vi "iWorx - Humidity.vi"() -> ()   [LabVIEW 2012]
uses:
  <vilib>/DAQmx/create/channels.llb/DAQmx Create Channel (AI-Voltage-Basic).vi
  <vilib>/DAQmx/read.llb/DAQmx Read (Analog 1D Wfm NChan 1Samp).vi
  vi.lib/iWorx/iWorx Set Points.ctl
panel:
  in  "Reset Scale":bool
  in  "Stop":bool
  in  "Log Info Button":bool
  in  "Set Up":bool
  in  "Channel":u16(ring) items=["Channel 1", "Channel 2"]
  in  "Pause Button":bool
  in  "Snapshot":bool
  out "Processed Signal":dbl(knob) caption="Relative Humidity" scale=0.0..100.0
  out "Waveform Chart":waveform(dbl)(graph)
  in  "Sample Timing":u16(ring)=200 items=["20Hz"=50, "5 Hz"=200, "2 Hz"=500, "1 Hz"=1000, ".5 Hz"=2000, ".2 Hz"=5000]
  in  "Clear Chart":bool
  in  "Open Log":bool
  in  "Rescale Y":bool
  out "Raw Signal":dbl(knob) scale=-5.0..5.0
  # "iWorx - Humidity - Data Logger"
  # "Sensor Input"
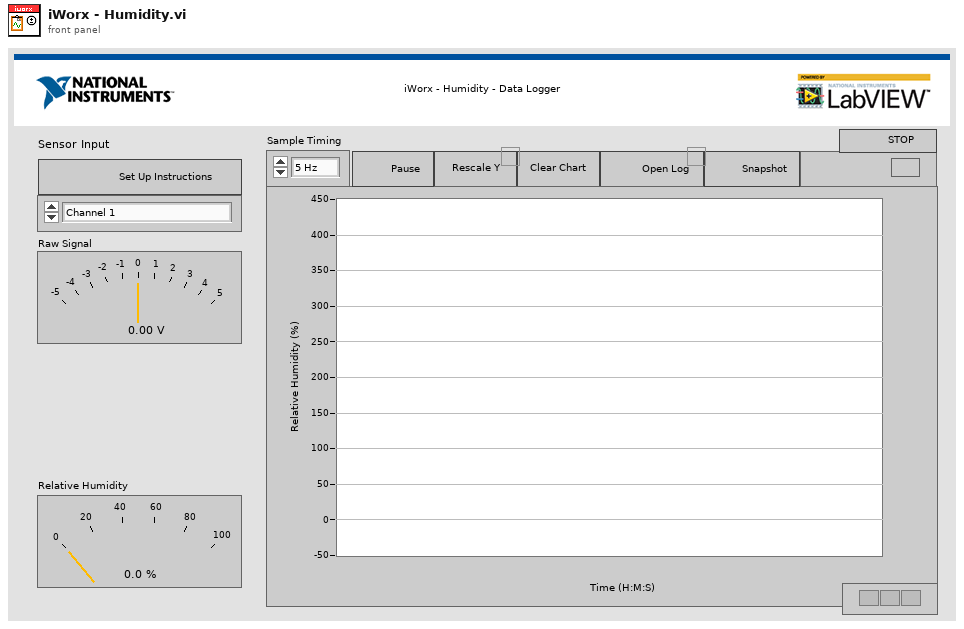
[diagram p1: front panel]
types:
  T1 = typedef "iWorx Set Points.ctl" = cluster{"SP1 Voltage":dbl, "SP1 Value":dbl, "SP2 Voltage":dbl, "SP2 Value":dbl}
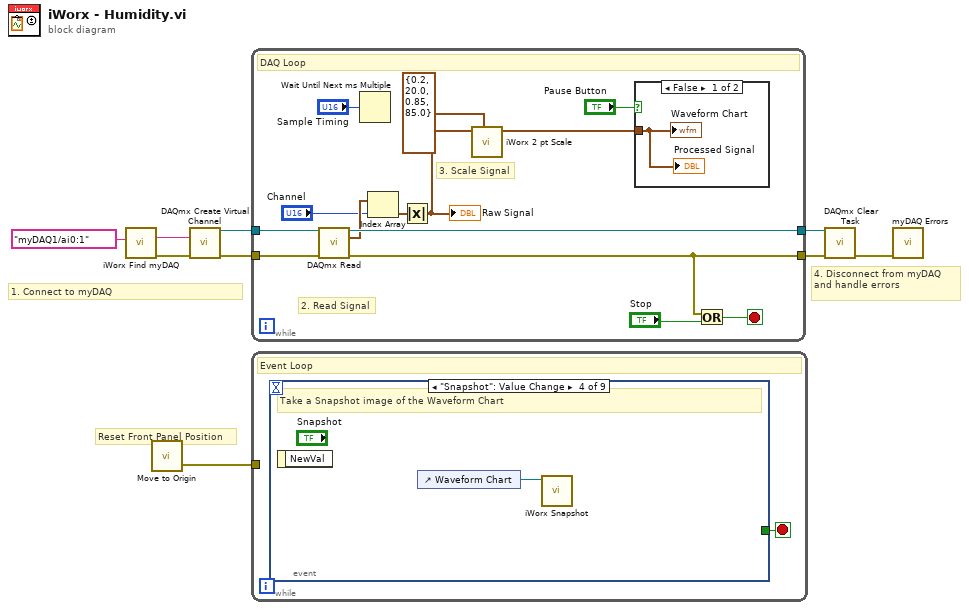
[diagram p0: block diagram]
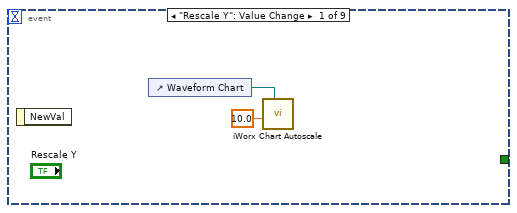
[diagram p2: hidden frame]
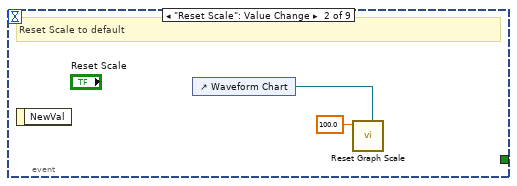
[diagram p3: hidden frame]
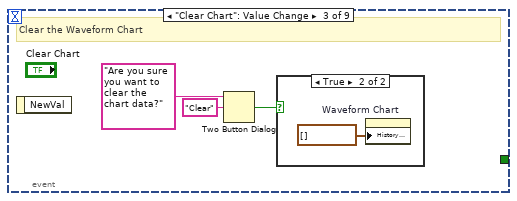
[diagram p4: hidden frame]
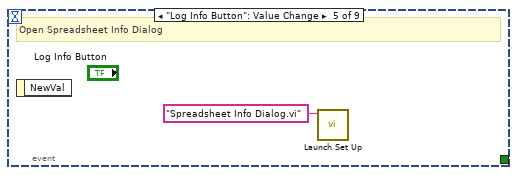
[diagram p6: hidden frame]
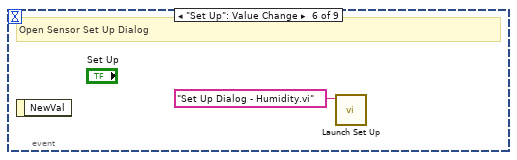
[diagram p7: hidden frame]
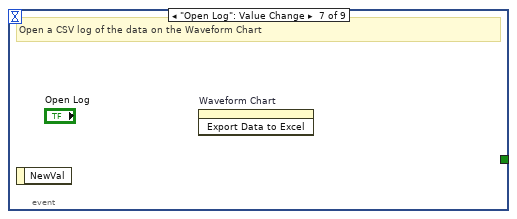
[diagram p8: hidden frame]
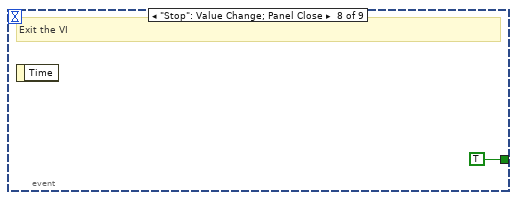
[diagram p9: hidden frame]
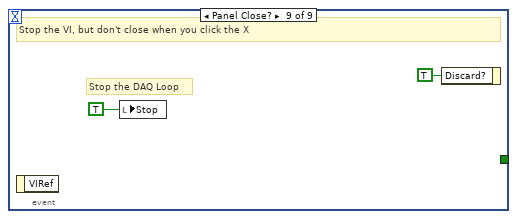
[diagram p10: hidden frame]
diagram:
  # "Reset Front Panel Position"
  # "4. Disconnect from myDAQ and handle errors"
  # "1. Connect to myDAQ"
  n1 = call "iWorx Find myDAQ.vi"("Preferred myDAQ (myDAQ1)"=tag "myDAQ1/ai0:1") -> ("Error Out"=w3:errorcluster, "DAQmx Physical Channel"=w4:tag)  [unwired: 6 in, 3 out]
  n2 = call "Move to Origin.vi"() -> ("Error Out"=w1:errorcluster)  [unwired: 3 in]
  n3 = call-poly <vilib>:"DAQmx Create Virtual Channel.vi"("physical channels"=w4, "error in"=w3) -> ("task out"=w7:refnum<k21>, "error out"=w6:errorcluster)  [unwired: 12 in]
  n4 = while {
    tunnel: w7 -> [w22]
    tunnel: [w21] -> w9
    tunnel: w6 -> [w20]
    tunnel: [w18] -> w8
    stop <- w19 stop-if-true
    # "3. Scale Signal"
    # "2. Read Signal"
    # "DAQ Loop"
    n5 = call-poly <vilib>:"DAQmx Read.vi"("task/channels in"=w22, "error in"=w20) -> ("task out"=w21:refnum<k21>, "data"=w16:waveform(dbl)[], "error out"=w18:errorcluster)  [unwired: 11 in]
    n6 = Wait Until Next ms Multiple(millisecond multiple="Sample Timing") -> ()  [unwired: 1 out]
    n7 = Index Array(array=w16, index="Channel") -> (element=w11:waveform(dbl))
    n8 = Absolute Value(x=w11) -> (abs(x)=w10:waveform(dbl))
    "Raw Signal" <- w10
    n9 = call "iWorx 2 pt Scale.vi"("Set Points"=T1 {"SP1 Voltage"=0.2, "SP1 Value"=20.0, "SP2 Voltage"=0.85, "SP2 Value"=85.0}, "Raw Waveform"=w10) -> ("Scaled Value"=w15:waveform(dbl))  [unwired: 7 in, 2 out]
    n10 = case shown="False" "Pause Button" {
      tunnel: w15 -> [w24 _]
      frame False {
        "Waveform Chart" <- w24
        "Processed Signal" <- w24
      }
      frame True {
        # "Do Not update controls"
      }
    }
    n11 = Or(x=w18, y="Stop") -> (x .or. y?=w19:bool)
  }
  n12 = while {
    tunnel: w1 -> [_]
    stop <- w25 stop-if-true
    # "Event Loop"
    n13 = event shown="[3] \"Snapshot\": Value Change" {
      selector: _ -> [_ _ _ _ _ _ _ _ _]
      dyn-events: _ -> [_ _ _ _ _ _ _ _ _]
      timeout: _ -> [_ _ _ _ _ _ _ _ _]
      tunnel: [_ _ _ _ _ _ _ TRUE _] -> w25
      event "Rescale Y": Value Change {
        n14 = event-data() -> ()  [unwired: 1 in, 1 out]
        n15 = control-ref of="Waveform Chart"() -> (w27:refnum<vi>)
        n16 = call "iWorx Chart Autoscale.vi"("Selection Chart"=w27, "Rounding Multiple (10)"=10.0 ("Rounding Multiple (1)")) -> ()  [unwired: 7 in, 3 out]
      }
      event "Reset Scale": Value Change {
        # "Reset Scale to default"
        n17 = event-data() -> ()  [unwired: 1 in, 1 out]
        n18 = control-ref of="Waveform Chart"() -> (w29:refnum<vi>)
        n19 = call "Reset Graph Scale.vi"("WaveformChart in"=w29, "Maximum (100)"=100.0) -> ()  [unwired: 9 in, 1 out]
      }
      event "Clear Chart": Value Change {
        # "Clear the Waveform Chart"
        n20 = event-data() -> ()  [unwired: 1 in, 1 out]
        n21 = Two Button Dialog(message="Are you sure you want to clear the chart data?", 2:"Clear" ("T button name (\"OK\")")) -> (T button?=w31:bool)  [unwired: 1 in]
        n22 = case shown="True" w31 {
          frame False {
          }
          frame True {
            n23 = property on="Waveform Chart" class="WFChart (strict)"("History Data"=waveform(dbl)[] []) -> ()  [unwired: 2 in, 2 out]
          }
        }
      }
      event "Snapshot": Value Change {
        # "Take a Snapshot image of the Waveform Chart"
        n24 = event-data() -> ()  [unwired: 1 in, 1 out]
        n25 = control-ref of="Waveform Chart"() -> (w34:refnum<vi>)
        n26 = call "iWorx Snapshot.vi"("WaveformChart in"=w34) -> ()  [unwired: 10 in, 1 out]
      }
      event "Log Info Button": Value Change {
        # "Open Spreadsheet Info Dialog"
        n27 = event-data() -> ()  [unwired: 1 in, 1 out]
        n28 = call "Launch Set Up.vi"("name or relative path"="Spreadsheet Info Dialog.vi") -> ()  [unwired: 9 in, 2 out]
      }
      event "Set Up": Value Change {
        # "Open Sensor Set Up Dialog"
        n29 = event-data() -> ()  [unwired: 1 in, 1 out]
        n30 = call "Launch Set Up.vi"("name or relative path"="Set Up Dialog - Humidity.vi") -> ()  [unwired: 9 in, 2 out]
      }
      event "Open Log": Value Change {
        # "Open a CSV log of the data on the Waveform Chart"
        n31 = event-data() -> ()  [unwired: 1 in, 1 out]
        n32 = invoke on="Waveform Chart" class="WFChart (strict)" method="Export Data to Excel"() -> ()  [unwired: 3 in, 3 out]
      }
      event "Stop": Value Change; Panel Close {
        # "Exit the VI"
        n33 = event-data() -> ()  [unwired: 1 in, 1 out]
      }
      event Panel Close? {
        # "Stop the DAQ Loop"
        # "Stop the VI, but don't close when you click the X"
        n34 = event-data() -> ()  [unwired: 1 in, 1 out]
        n35 = local write "Stop"(TRUE ("stop")) -> ()
        n36 = event-data("Discard?"=TRUE) -> ()  [unwired: 1 in, 1 out]
      }
    }
  }
  n37 = call <vilib>:"DAQmx Clear Task.vi"("task in"=w9, "error in"=w8) -> ("error out"=w5:errorcluster)  [unwired: 13 in]
  n38 = call "myDAQ Errors.vi"("error in (no error)"=w5) -> ()  [unwired: 10 in, 1 out]
